vi "get_cap.vi"() -> (3 "return type":string[](array[string]))   [LabVIEW 2019]
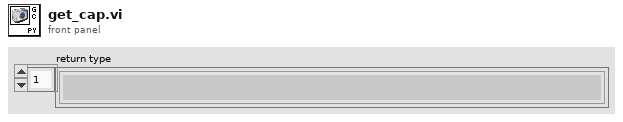
[diagram p1: front panel]
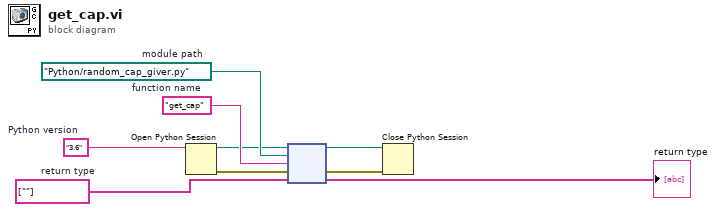
[diagram p0: block diagram]
diagram:
  w7 = string[] [""]  # return type
  w5 = "get_cap"  # function name
  w8 = path "Python/random_cap_giver.py"  # module path
  w2 = "3.6"  # Python version
  n1 = Open Python Session(python version=w2) -> (session out=w1:refnum<k35>, error out=w4:errorcluster)  [unwired: 2 in]
  n2 = node ("Python Node")(w1, w8, w5, w4, w7) -> (w3:refnum<k35>, w6:errorcluster, →"return type":string[])  [unwired: 2 out]
  n3 = Close Python Session(session in=w3, error in=w6) -> ()  [unwired: 1 out]
